vi "Program19.vi"() -> ()   [LabVIEW 2020]
uses:
  <vilib>/Utility/error.llb/DialogType.ctl
  <vilib>/Analysis/baseanly.llb/Mean (DBL).vi
  <vilib>/Utility/file.llb/Read Delimited Spreadsheet (DBL).vi
  <vilib>/Analysis/NI_AALBase.lvlib
  <vilib>/gmath/NI_Gmath.lvlib
panel:
  in  "Manual":bool
  in  "REF3":dbl=1000.0 format="%#.0f"
  in  "REF2":dbl=1000.0 format="%#.0f"
  in  "REF1":dbl=1000.0 format="%#.0f"
  out "REF":dbl[](array[numeric])
  out "INT4":dbl[](array[numeric])
  out "S1+ S2 = Sx + Sy":bool
  out "Filenames":string[](array[string])
  out "INT3":dbl[](array[numeric])
  out "INT2":dbl[](array[numeric])
  out "INT1":dbl[](array[numeric])
  out "Wczytane":dbl[][](array[numeric])
  out "Loaded data":path
  out "Calibration":path
  out "Saved file":path
  in  "Save data":bool
  out "A":dbl[](array[numeric]) format="%#.0f"
  out "B":dbl[](array[numeric]) format="%#.0f"
  out "Sy":dbl[](array[numeric]) format="%#.0f"
  out "Sx":dbl[](array[numeric]) format="%#.0f"
  out "S2":dbl[](array[numeric]) format="%#.0f"
  out "S1":dbl[](array[numeric]) format="%#.0f"
  out "YY":dbl[][](array[numeric])
  out "XX":dbl[][](array[numeric])
  out "Data loaded":bool
  out "Calibration loaded":bool
  in  "0_45_90/45_90_135":bool
  in  "Run":bool
  in  "Stop":bool
  in  "Loda data":bool
  in  "Load calibration":bool
  in  "anisotropic?":bool
  in  "Poisson":dbl=0.33 min=0.0 max=1.0 step=0.01 format="%#_2g"
  in  "Young":dbl=0.22 min=0.0 max=1.0 step=0.01 format="%#_2g"
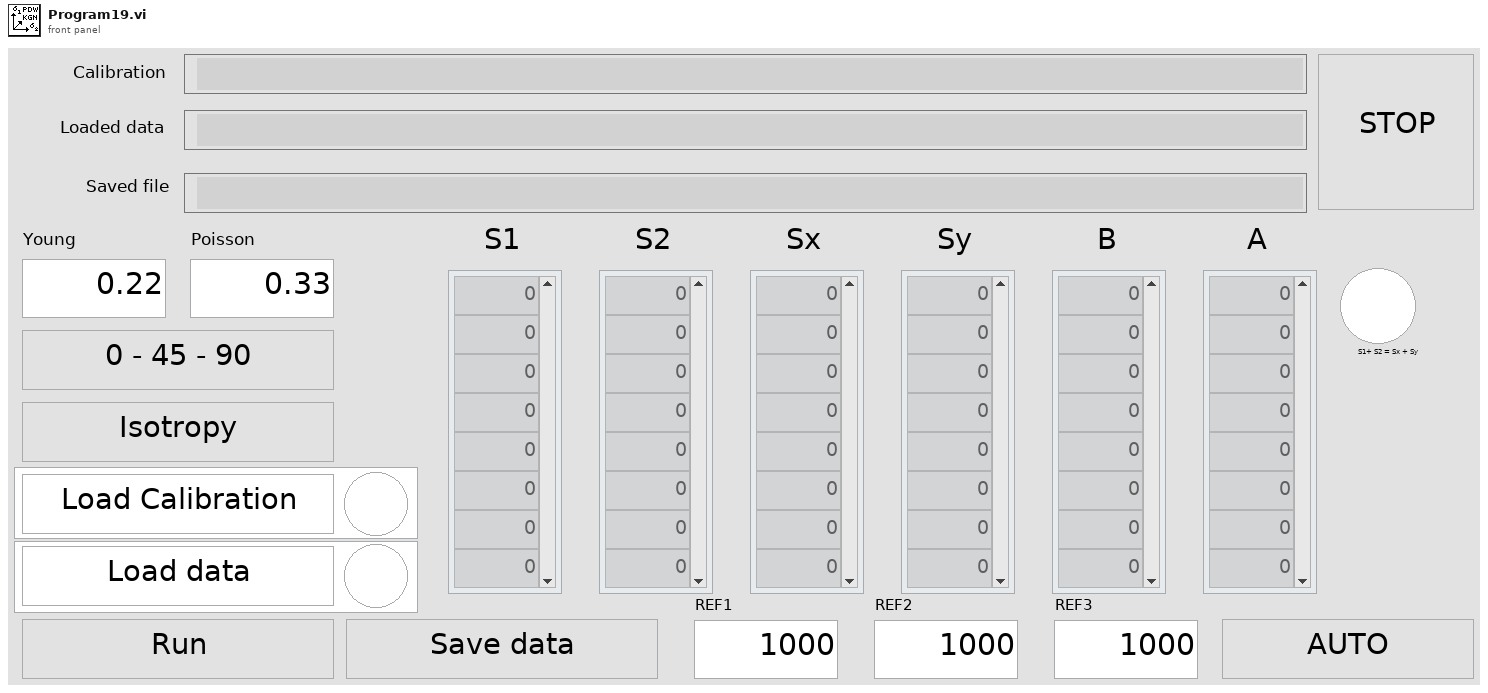
[diagram p1: front panel]
types:
  T1 = enum8{"Enabled", "Disabled", "Disabled and Grayed Out"}
  T2 = typedef "DialogType.ctl" = u16
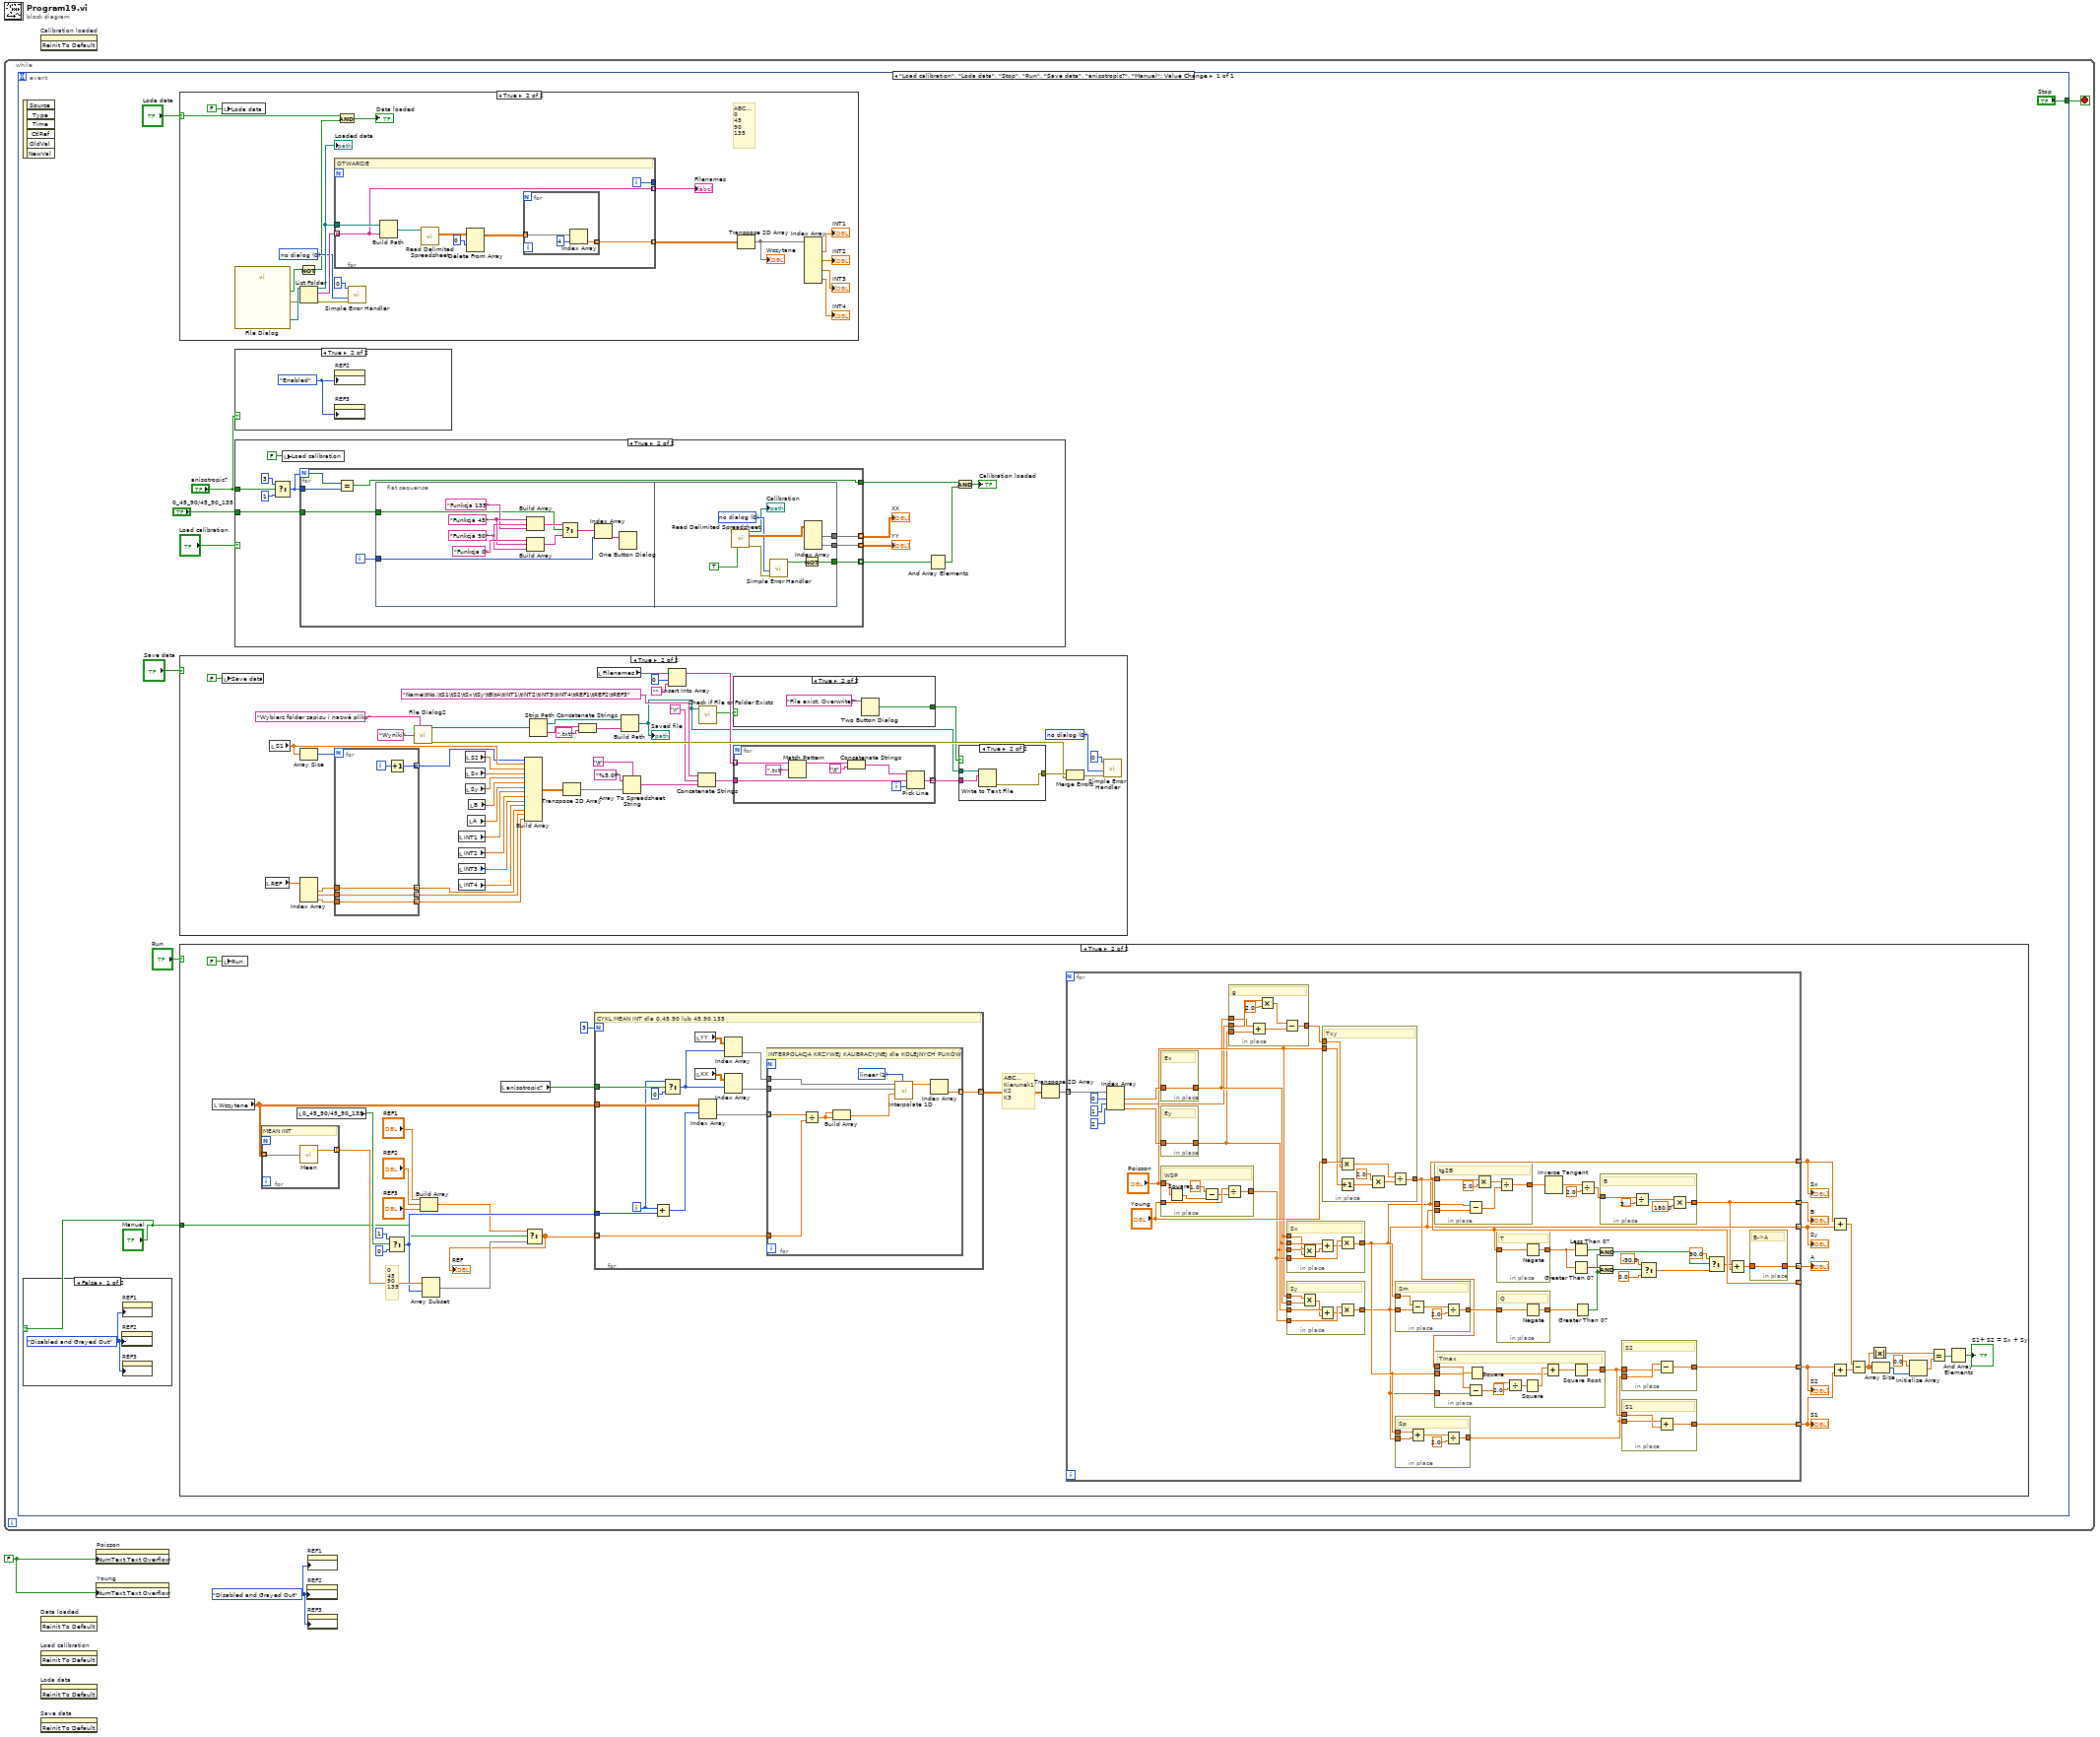
[diagram p0: block diagram]
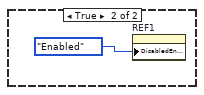
[diagram p2: hidden frame]
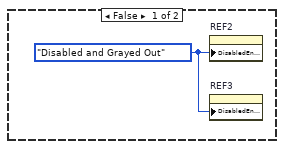
[diagram p3: hidden frame]
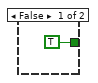
[diagram p5: hidden frame]
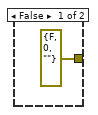
[diagram p6: hidden frame]
diagram:
  w1 = T1."Disabled and Grayed Out" ("Disabled")
  w2 = FALSE ("Numeric Text.Text Overflow")
  n1 = while {
    stop <- w3 stop-if-true
    n2 = event shown="[0] \"Load calibration\", \"Loda data\", \"Stop\", \"Run\", \"Save data\", \"anisotropic?\", \"Manual\": Value Change" {
      selector: _ -> [_]
      dyn-events: _ -> [_]
      timeout: _ -> [_]
      tunnel: ["Stop"] -> w3
      event "Load calibration", "Loda data", "Stop", "Run", "Save data", "anisotropic?", "Manual": Value Change {
        n3 = event-data() -> ()  [unwired: 1 in, 6 out]
        n4 = case shown="False" "Manual" {
          frame False {
            w12 = T1."Disabled and Grayed Out" ("Disabled")
            n5 = property on="REF2" class="DigNum (strict)"("DisabledEnum"=w12) -> ()  [unwired: 2 in, 2 out]
            n6 = property on="REF1" class="DigNum (strict)"("DisabledEnum"=w12) -> ()  [unwired: 2 in, 2 out]
            n7 = property on="REF3" class="DigNum (strict)"("DisabledEnum"=w12) -> ()  [unwired: 2 in, 2 out]
          }
          frame True {
            n8 = property on="REF1" class="DigNum (strict)"("DisabledEnum"=T1."Enabled" ("Disabled")) -> ()  [unwired: 2 in, 2 out]
          }
        }
        n9 = case shown="True" "Loda data" {
          selector: "Loda data" -> [_ w271]
          frame False {
          }
          frame True {
            w272 = T2 0 items=["no dialog", "OK message", "continue or stop message", "OK message + warnings", "continue/stop + warnings"] ("type of dialog (OK msg:1)")
            # "ABC...\n0\n45\n90\n135"
            n10 = local write "Loda data"(FALSE ("Boolean")) -> ()
            n11 = call "File Dialog"() -> ("selected path"=w278:path, "cancelled"=w270:bool, "error out"=w274:errorcluster)  [unwired: 12 in, 1 out]
            n12 = Not(x=w270) -> (.not. x?=w269:bool)
            n13 = List Folder(path=w278, error in=w274) -> (path out=w279:path, filenames=w280:string[], error out=w273:errorcluster)  [unwired: 2 in, 1 out]
            "Loaded data" <- w279
            n14 = for {
              tunnel: w280 -> [w281] mode=indexing
              tunnel: w279 -> [w288]
              tunnel: [w283] -> w277 mode=indexing
              tunnel: [w282] -> _
              tunnel: [w281] -> w267 mode=indexing
              i -> [w282]
              # "OTWARCIE"
              n15 = Build Path(base path=w288, name or relative path=w281) -> (appended path=w287:path)
              n16 = call-poly <vilib>:"Read Delimited Spreadsheet.vi"("file path (dialog if empty)"=w287) -> ("all rows"=w286:dbl[][])  [unwired: 9 in, 5 out]
              n17 = Delete From Array(array=w286, index (row)=0) -> (array with subset deleted=w284:dbl[][])  [unwired: 2 in, 1 out]
              n18 = for {
                tunnel: w284 -> [w290] mode=indexing
                tunnel: [w289] -> w283 mode=indexing
                n19 = Index Array(array=w290, index=4) -> (element=w289:dbl)
              }
            }
            "Filenames" <- w267
            n20 = And(x=w271, y=w269) -> (x .and. y?=→"Data loaded":bool)
            n21 = call <vilib>:"Simple Error Handler.vi"("error code (no error:0)"=0, "type of dialog (OK msg:1)"=w272, "error in (no error)"=w273) -> ()  [unwired: 2 in, 5 out]
            n22 = Transpose 2D Array(2D array=w277) -> (transposed array=w266:dbl[][])
            "Wczytane" <- w266
            n23 = Index Array(array=w266) -> (element #1=→"INT1":dbl[], element #2=→"INT2":dbl[], element #3=→"INT3":dbl[], element #4=→"INT4":dbl[])  [unwired: 8 in]
          }
        }
        n24 = case shown="True" "Save data" {
          frame False {
          }
          frame True {
            w57 = T2 0 items=["no dialog", "OK message", "continue or stop message", "OK message + warnings", "continue/stop + warnings"] ("type of dialog (OK msg:1)")
            n25 = local write "Save data"(FALSE ("Save data")) -> ()
            n26 = local read "REF"() -> (w22:dbl[])
            n27 = local read "S1"() -> (w54:dbl[])
            n28 = Array Size(array=w54) -> (size(s)=w53:i32)
            n29 = Index Array(array=w22) -> (element #1=w21:dbl, element #2=w20:dbl, element #3=w19:dbl)  [unwired: 3 in]
            n30 = for {
              N: w53 -> [_]
              tunnel: [w82] -> w52 mode=indexing
              tunnel: w21 -> [w81]
              tunnel: w20 -> [w80]
              tunnel: w19 -> [w79]
              tunnel: [w81] -> w18 mode=indexing
              tunnel: [w80] -> w17 mode=indexing
              tunnel: [w79] -> w16 mode=indexing
              i -> [w83]
              n31 = Increment(x=w83) -> (x+1=w82:i32)
            }
            n32 = call "File Dialog2"("prompt"="Wybierz folder zapisu i nazwê pliku", "default name"="Wyniki") -> ("selected path"=w46:path, "error out"=w49:errorcluster)  [unwired: 10 in, 2 out]
            n33 = local read "INT1"() -> (w41:dbl[])
            n34 = local read "INT2"() -> (w40:dbl[])
            n35 = local read "INT3"() -> (w39:dbl[])
            n36 = local read "INT4"() -> (w23:dbl[])
            n37 = local read "S2"() -> (w63:dbl[])
            n38 = local read "Sx"() -> (w62:dbl[])
            n39 = local read "Sy"() -> (w61:dbl[])
            n40 = local read "A"() -> (w59:dbl[])
            n41 = local read "B"() -> (w60:dbl[])
            n42 = Build Array(w52, w54, w63, w62, w61, w60, w59, w41, w40, w39, w23, w18, w17, w16) -> (w35:dbl[][])
            n43 = Strip Path(path=w46) -> (stripped path=w45:path, name=w44:string)
            n44 = Transpose 2D Array(2D array=w35) -> (transposed array=w34:dbl[][])
            n45 = Concatenate Strings(w44, ".txt" ("string")) -> (w42:string)
            n46 = local read "Filenames"() -> (w31:string[])
            n47 = Build Path(base path=w45, name or relative path=w42) -> (appended path=w27:path)
            "Saved file" <- w27
            n48 = Array To Spreadsheet String(delimiter (Tab)="\t", array=w34, 3:"%5.0f" ("format string")) -> (spreadsheet string=w33:string)
            n49 = Insert Into Array(array=w31, index=0, new element="") -> (w28:string[])
            n50 = Concatenate Strings("Name\tNo.\tS1\tS2\tSx\tSy\tB\tA\tINT1\tINT2\tINT3\tINT4\tREF1\tREF2\tREF3" ("string"), "\r", w33) -> (w36:string)
            n51 = call <vilib>:"Check if File or Folder Exists.vi"("path"=w27) -> ("file or folder exists?"=w25:bool)  [unwired: 8 in, 2 out]
            n52 = case shown="True" w25 {
              tunnel: [TRUE ("T button?") w65] -> w24
              frame False {
              }
              frame True {
                n53 = Two Button Dialog(message="File exist. Overwrite?") -> (T button?=w65:bool)  [unwired: 2 in]
              }
            }
            n54 = for {
              tunnel: w28 -> [w74] mode=indexing
              tunnel: w36 -> [w78]
              tunnel: [w77] -> w32 mode=indexing
              i -> [w75]
              n55 = Match Pattern(string=w74, regular expression=".txt") -> (before substring=w72:string)  [unwired: 1 in, 3 out]
              n56 = Concatenate Strings(w72, "\t") -> (w71:string)
              n57 = Pick Line(string ("")=w71, multi-line string=w78, line index=w75) -> (output string=w77:string)
            }
            n58 = case shown="True" w24 {
              tunnel: [errorcluster {"status"=FALSE, "code"=0, "source"=""} ("error out") w70] -> w50
              tunnel: w32 -> [_ w69]
              tunnel: w27 -> [_ w68]
              frame False {
              }
              frame True {
                n59 = Write to Text File(file (use dialog)=w68, text=w69) -> (error out=w70:errorcluster)  [unwired: 2 in, 2 out]
              }
            }
            n60 = Merge Errors(w50, w49) -> (w48:errorcluster)
            n61 = call <vilib>:"Simple Error Handler.vi"("error code (no error:0)"=0, "type of dialog (OK msg:1)"=w57, "error in (no error)"=w48) -> ()  [unwired: 2 in, 5 out]
          }
        }
        n62 = case shown="True" "Run" {
          tunnel: "Manual" -> [_ w85]
          frame False {
          }
          frame True {
            # "ABC...\nKierunek1\nK2\nK3"
            # "0\n45\n90\n135"
            n63 = local read "Wczytane"() -> (w102:dbl[][])
            n64 = local write "Run"(FALSE ("Boolean")) -> ()
            n65 = for {
              tunnel: w102 -> [w141] mode=indexing
              tunnel: [w140] -> w101 mode=indexing
              # "MEAN INT"
              n66 = call-poly <vilib>:"Mean.vi"("X"=w141) -> ("mean"=w140:dbl)  [unwired: 1 out]
            }
            n67 = local read "0_45_90/45_90_135"() -> (w93:bool)
            n68 = Select(t=1, s=w93, f=0) -> (s? t:f=w94:i32)
            n69 = Build Array("REF1", "REF2", "REF3") -> (w87:dbl[])
            n70 = Array Subset(array=w101, index=w94) -> (w86:dbl[])  [unwired: 1 in]
            n71 = local read "anisotropic?"() -> (w92:bool)
            n72 = Select(t=w87, s=w85, f=w86) -> (s? t:f=w84:dbl[])
            "REF" <- w84
            n73 = for {
              N: 3 -> [_]
              tunnel: w84 -> [w130] mode=indexing
              tunnel: w102 -> [w127]
              tunnel: [w129] -> w97 mode=indexing
              tunnel: w94 -> [w122]
              tunnel: w92 -> [w120]
              i -> [w119]
              # "CYKL MEAN INT dla 0,45,90 lub 45,90,135"
              n74 = Add(x=w119, y=w122) -> (x+y=w121:i32)
              n75 = Select(t=w119, s=w120, f=0) -> (s? t:f=w118:i32)
              n76 = local read "YY"() -> (w125:dbl[][])
              n77 = local read "XX"() -> (w126:dbl[][])
              n78 = Index Array(array=w127, index (row)=w121) -> (element=w128:dbl[])  [unwired: 1 in]
              n79 = Index Array(array=w125, index (row)=w118) -> (element=w123:dbl[])  [unwired: 1 in]
              n80 = Index Array(array=w126, index (row)=w118) -> (element=w124:dbl[])  [unwired: 1 in]
              n81 = for {
                tunnel: w130 -> [w135]
                tunnel: [w133] -> w129 mode=indexing
                tunnel: w128 -> [w136] mode=indexing
                tunnel: w124 -> [w132]
                tunnel: w123 -> [w131]
                w139 = 1 items=["nearest", "linear", "spline", "cubic Hermite", "Lagrange"] ("method")
                # "INTERPOLACJA KRZYWEJ KALIBRACYJNEJ dla KOLEJNYCH PLIKÓW"
                n82 = Divide(x=w136, y=w135) -> (x/y=w138:dbl)
                n83 = Build Array(w138, w138) -> (w137:dbl[])
                n84 = call <vilib>:"Interpolate 1D.vi"("method"=w139, "xi"=w137, "X"=w132, "Y"=w131) -> ("yi"=w134:dbl[])  [unwired: 5 in, 2 out]
                n85 = Index Array(array=w134) -> (element=w133:dbl)  [unwired: 1 in]
              }
            }
            n86 = Transpose 2D Array(2D array=w97) -> (transposed array=w116:dbl[][])
            n87 = for {
              tunnel: [w181] -> w107 mode=indexing
              tunnel: [w180] -> w108 mode=indexing
              tunnel: w116 -> [w169] mode=indexing
              tunnel: [w164] -> w106 mode=indexing
              tunnel: [w165] -> w105 mode=indexing
              tunnel: [w166] -> _ mode=indexing
              tunnel: [w152] -> w103 mode=indexing
              tunnel: [w145] -> w104 mode=indexing
              n88 = Index Array(array=w169, index #1=0 ("index"), index #2=1 ("index"), index #3=2 ("index")) -> (element #1=w177:dbl, element #2=w142:dbl, element #3=w178:dbl)
              n89 = in-place {
                in-place-border: w177 -> [w193]
                in-place-border: [w193] -> w144
                # "Ex"
              }
              n90 = in-place {
                in-place-border: w178 -> [w192]
                in-place-border: [w192] -> w143
                # "Ey"
              }
              n91 = in-place {
                in-place-border: "Young" -> [w239]
                in-place-border: "Poisson" -> [w237]
                in-place-border: [w234] -> w168
                # "WSP"
                n92 = Square(x=w237) -> (x^2=w236:dbl)
                n93 = Subtract(x=1.0, y=w236) -> (x-y=w235:dbl)
                n94 = Divide(x=w239, y=w235) -> (x/y=w234:dbl)
              }
              n95 = in-place {
                in-place-border: w142 -> [w246]
                in-place-border: w144 -> [w244]
                in-place-border: w143 -> [w243]
                in-place-border: [w240] -> w167
                # "g"
                n96 = Add(x=w244, y=w243) -> (x+y=w241:dbl)
                n97 = Multiply(x=w246, y=2.0) -> (x*y=w242:dbl)
                n98 = Subtract(x=w242, y=w241) -> (x-y=w240:dbl)
              }
              n99 = in-place {
                in-place-border: w168 -> [w253]
                in-place-border: w144 -> [w252]
                in-place-border: "Poisson" -> [w251]
                in-place-border: w143 -> [w250]
                in-place-border: [w247] -> w165
                # "Sx"
                n100 = Multiply(x=w251, y=w250) -> (x*y=w249:dbl)
                n101 = Add(x=w252, y=w249) -> (x+y=w248:dbl)
                n102 = Multiply(x=w253, y=w248) -> (x*y=w247:dbl)
              }
              n103 = in-place {
                in-place-border: w168 -> [w233]
                in-place-border: w143 -> [w232]
                in-place-border: "Poisson" -> [w231]
                in-place-border: w144 -> [w230]
                in-place-border: [w227] -> w164
                # "Sy"
                n104 = Multiply(x=w231, y=w230) -> (x*y=w229:dbl)
                n105 = Add(x=w232, y=w229) -> (x+y=w228:dbl)
                n106 = Multiply(x=w233, y=w228) -> (x*y=w227:dbl)
              }
              n107 = in-place {
                in-place-border: "Young" -> [w261]
                in-place-border: w167 -> [w260]
                in-place-border: "Poisson" -> [w255]
                in-place-border: [w254] -> w166
                # "Txy"
                n108 = Multiply(x=w261, y=w260) -> (x*y=w259:dbl)
                n109 = Increment(x=w255) -> (x+1=w256:dbl)
                n110 = Multiply(x=2.0, y=w256) -> (x*y=w258:dbl)
                n111 = Divide(x=w259, y=w258) -> (x/y=w254:dbl)
              }
              n112 = in-place {
                in-place-border: w165 -> [w221]
                in-place-border: w164 -> [w220]
                in-place-border: [w217] -> w179
                # "Sm"
                n113 = Subtract(x=w221, y=w220) -> (x-y=w218:dbl)
                n114 = Divide(x=w218, y=2.0) -> (x/y=w217:dbl)
              }
              n115 = in-place {
                in-place-border: w165 -> [w226]
                in-place-border: w164 -> [w225]
                in-place-border: [w222] -> w175
                # "Sp"
                n116 = Add(x=w226, y=w225) -> (x+y=w223:dbl)
                n117 = Divide(x=w223, y=2.0) -> (x/y=w222:dbl)
              }
              n118 = in-place {
                in-place-border: w166 -> [w199]
                in-place-border: w165 -> [w197]
                in-place-border: w164 -> [w196]
                in-place-border: [w194] -> w151
                # "tg2B"
                n119 = Subtract(x=w197, y=w196) -> (x-y=w195:dbl)
                n120 = Multiply(x=w199, y=2.0) -> (x*y=w198:dbl)
                n121 = Divide(x=w198, y=w195) -> (x/y=w194:dbl)
              }
              n122 = in-place {
                in-place-border: w165 -> [w210]
                in-place-border: w164 -> [w209]
                in-place-border: w166 -> [w208]
                in-place-border: [w207] -> w176
                # "Tmax"
                n123 = Subtract(x=w210, y=w209) -> (x-y=w213:dbl)
                n124 = Square(x=w208) -> (x^2=w214:dbl)
                n125 = Divide(x=w213, y=2.0) -> (x/y=w211:dbl)
                n126 = Square(x=w211) -> (x^2=w215:dbl)
                n127 = Add(x=w215, y=w214) -> (x+y=w216:dbl)
                n128 = Square Root(x=w216) -> (sqrt(x)=w207:dbl)
              }
              n129 = in-place {
                in-place-border: w166 -> [w189]
                in-place-border: [w188] -> w163
                # "T"
                n130 = Negate(x=w189) -> (-x=w188:dbl)
              }
              n131 = in-place {
                in-place-border: w179 -> [w191]
                in-place-border: [w190] -> w162
                # "Q"
                n132 = Negate(x=w191) -> (-x=w190:dbl)
              }
              n133 = Inverse Tangent(1:w151) -> (0:w149:dbl)
              n134 = Less Than 0?(x=w163) -> (x < 0?=w156:bool)
              n135 = Greater Than 0?(x=w163) -> (x > 0?=w161:bool)
              n136 = Greater Than 0?(x=w162) -> (x > 0?=w157:bool)
              n137 = Divide(x=w149, y=2.0) -> (x/y=w148:dbl)
              n138 = And(x=w156, y=w157) -> (x .and. y?=w155:bool)
              n139 = And(x=w161, y=w157) -> (x .and. y?=w159:bool)
              n140 = in-place {
                in-place-border: w148 -> [w186]
                in-place-border: [w182] -> w145
                # "B"
                n141 = Divide(x=w186, y=3.141592653589793) -> (x/y=w184:dbl)
                n142 = Multiply(x=w184, y=180.0) -> (x*y=w182:dbl)
              }
              n143 = in-place {
                in-place-border: w175 -> [w203]
                in-place-border: w176 -> [w202]
                in-place-border: [w201] -> w181
                # "S2"
                n144 = Subtract(x=w203, y=w202) -> (x-y=w201:dbl)
              }
              n145 = in-place {
                in-place-border: w175 -> [w206]
                in-place-border: w176 -> [w205]
                in-place-border: [w204] -> w180
                # "S1"
                n146 = Add(x=w206, y=w205) -> (x+y=w204:dbl)
              }
              n147 = Select(t=-90.0, s=w159, f=0.0) -> (s? t:f=w154:dbl)
              n148 = Select(t=90.0, s=w155, f=w154) -> (s? t:f=w147:dbl)
              n149 = Add(x=w147, y=w145) -> (x+y=w146:dbl)
              n150 = in-place {
                in-place-border: w146 -> [w187]
                in-place-border: [w187] -> w152
                # "B->A"
              }
            }
            "S1" <- w108
            "B" <- w104
            "A" <- w103
            "Sy" <- w106
            "S2" <- w107
            "Sx" <- w105
            n151 = Add(x=w105, y=w106) -> (x+y=w115:dbl[])
            n152 = Add(x=w107, y=w108) -> (x+y=w114:dbl[])
            n153 = Subtract(x=w115, y=w114) -> (x-y=w113:dbl[])
            n154 = Absolute Value(x=w113) -> (abs(x)=w110:dbl[])
            n155 = Array Size(array=w113) -> (size(s)=w111:i32)
            n156 = Initialize Array(0.0 ("element"), w111) -> (w109:dbl[])
            n157 = Equal?(x=w110, y=w109) -> (x = y?=w96:bool[])
            n158 = And Array Elements(Boolean array=w96) -> (logical AND=→"S1+ S2 = Sx + Sy":bool)
          }
        }
        n159 = case shown="True" "anisotropic?" {
          frame False {
            w14 = T1."Disabled and Grayed Out" ("Disabled")
            n160 = property on="REF2" class="DigNum (strict)"("DisabledEnum"=w14) -> ()  [unwired: 2 in, 2 out]
            n161 = property on="REF3" class="DigNum (strict)"("DisabledEnum"=w14) -> ()  [unwired: 2 in, 2 out]
          }
          frame True {
            w15 = T1."Enabled" ("Disabled")
            n162 = property on="REF2" class="DigNum (strict)"("DisabledEnum"=w15) -> ()  [unwired: 2 in, 2 out]
            n163 = property on="REF3" class="DigNum (strict)"("DisabledEnum"=w15) -> ()  [unwired: 2 in, 2 out]
          }
        }
        n164 = case shown="True" "Load calibration" {
          tunnel: "anisotropic?" -> [_ w293]
          tunnel: "0_45_90/45_90_135" -> [_ w292]
          frame False {
          }
          frame True {
            n165 = Select(t=3, s=w293, f=1) -> (s? t:f=w296:i32)
            n166 = local write "Load calibration"(FALSE ("Load calibration")) -> ()
            n167 = for {
              N: w296 -> [w307]
              tunnel: w292 -> [w310]
              tunnel: [w309] -> w300 mode=indexing
              tunnel: [w308] -> w298
              tunnel: w296 -> [w306]
              tunnel: [w305] -> w295 mode=indexing
              tunnel: [w304] -> w294 mode=indexing
              i -> [w311]
              n168 = Equal?(x=w307, y=w306) -> (x = y?=w308:bool)
              n169 = flat-sequence {
                tunnel: w311 -> [w312]
                tunnel: w310 -> [w314]
                tunnel: [w325] -> w309
                tunnel: [w324] -> w305
                tunnel: [w323] -> w304
                frame #0 {
                  w318 = "Funkcja 90"
                  w319 = "Funkcja 45"
                  n170 = Build Array(w319, w318, "Funkcja 135") -> (w316:string[])
                  n171 = Build Array("Funkcja 0", w319, w318) -> (w315:string[])
                  n172 = Select(t=w316, s=w314, f=w315) -> (s? t:f=w313:string[])
                  n173 = Index Array(array=w313, index=w312) -> (element=w320:string)
                  n174 = One Button Dialog(message=w320) -> ()  [unwired: 1 in, 1 out]
                }
                frame #1 {
                  w328 = T2 0 items=["no dialog", "OK message", "continue or stop message", "OK message + warnings", "continue/stop + warnings"] ("type of dialog (OK msg:1)")
                  n175 = call-poly <vilib>:"Read Delimited Spreadsheet.vi"("transpose? (F)"=TRUE) -> ("new file path (Not A Path if cancelled)"=→"Calibration":path, "all rows"=w329:dbl[][], "error out"=w330:errorcluster)  [unwired: 9 in, 3 out]
                  n176 = call <vilib>:"Simple Error Handler.vi"("type of dialog (OK msg:1)"=w328, "error in (no error)"=w330) -> ("error?"=w326:bool)  [unwired: 3 in, 4 out]
                  n177 = Not(x=w326) -> (.not. x?=w325:bool)
                  n178 = Index Array(array=w329) -> (element #1=w324:dbl[], element #2=w323:dbl[])  [unwired: 4 in]
                }
              }
            }
            "XX" <- w295
            "YY" <- w294
            n179 = And Array Elements(Boolean array=w300) -> (logical AND=w299:bool)
            n180 = And(x=w298, y=w299) -> (x .and. y?=→"Calibration loaded":bool)
          }
        }
      }
    }
  }
  n181 = invoke on="Calibration loaded" class="Bool (strict)" method="Reinit To Default"() -> ()  [unwired: 3 in, 3 out]
  n182 = invoke on="Data loaded" class="Bool (strict)" method="Reinit To Default"() -> ()  [unwired: 3 in, 3 out]
  n183 = invoke on="Load calibration" class="Bool (strict)" method="Reinit To Default"() -> ()  [unwired: 3 in, 3 out]
  n184 = invoke on="Loda data" class="Bool (strict)" method="Reinit To Default"() -> ()  [unwired: 3 in, 3 out]
  n185 = invoke on="Save data" class="Bool (strict)" method="Reinit To Default"() -> ()  [unwired: 3 in, 3 out]
  n186 = property on="Poisson" class="DigNum (strict)"("NumText.Text Overflow"=w2) -> ()  [unwired: 2 in, 2 out]
  n187 = property on="Young" class="DigNum (strict)"("NumText.Text Overflow"=w2) -> ()  [unwired: 2 in, 2 out]
  n188 = property on="REF2" class="DigNum (strict)"("DisabledEnum"=w1) -> ()  [unwired: 2 in, 2 out]
  n189 = property on="REF1" class="DigNum (strict)"("DisabledEnum"=w1) -> ()  [unwired: 2 in, 2 out]
  n190 = property on="REF3" class="DigNum (strict)"("DisabledEnum"=w1) -> ()  [unwired: 2 in, 2 out]
